vi "GT Get Ext Ad Voltage.vi"(7 "pValue":dbl[](array[numeric]), 8 "error in (no error)":errorcluster caption="错误输入（无错误）", 9 "chn":i16, 10 "mdl":i16, 11 "cardNum":i16) -> (0 "error out":errorcluster caption="错误输出", 3 "function return":i16, 5 "pValue out":dbl[](array[numeric]))   [LabVIEW 2014, in "gts.lvlib"]
doc: "GT_API GT_GetExtAdVoltage(short cardNum,short mdl,short chn,double *pValue);"
uses:
  gts.lvlib
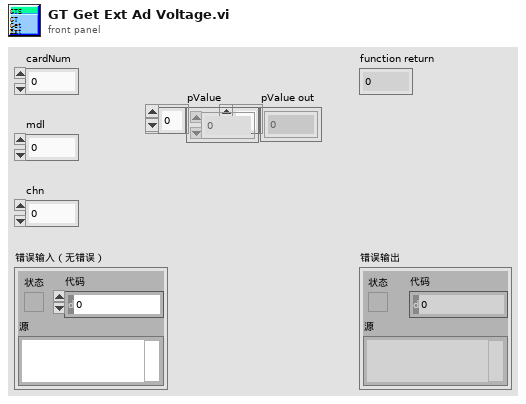
[diagram p1: front panel]
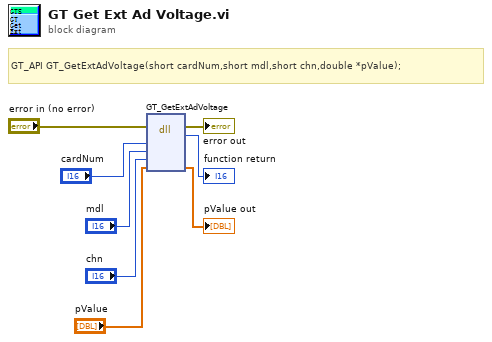
[diagram p0: block diagram]
diagram:
  # "GT_API GT_GetExtAdVoltage(short cardNum,short mdl,short chn,double *pValue);"
  n1 = dll-call lib="PTH2habs D固高科技资料GTS控制卡GTS卡18年上半年资料dllVC32bit\nmulti_cardgts.*" fn="GT_GetExtAdVoltage"(error in="error in (no error)", "cardNum"="cardNum", "mdl"="mdl", "chn"="chn", "pValue"="pValue") -> (error out=→"error out":errorcluster, "返回类型"=→"function return":i16, "pValue"=→"pValue out":dbl[])  [unwired: 5 in, 1 out]
